vi "Execute Tests.vi"(8 "error in (no error)":errorcluster, 10 "Tests":string[](array[string]), 11 "Execution UI In":refnum<class "Execution UI.lvclass">) -> (0 "error out":errorcluster, 3 "Execution UI Out":refnum<class "Execution UI.lvclass">)   [LabVIEW 2020, in "Execution UI.lvclass"]
uses:
  Execution UI.lvclass
  TypeDefs/Execution State.ctl
  Execution UI.lvclass/Execution UI.ctl
  LUnit Test Suite.lvclass
  C:/git/astemes-lunit/source/Runnable.lvclass
  Framework/Plugin/Plugin.lvclass
  Framework/Test Runner/Test Runner.lvclass
  Result Model by Reference/Result Model by Reference.lvclass
  C:/git/astemes-lunit/source/LUnit Test Suite.lvclass
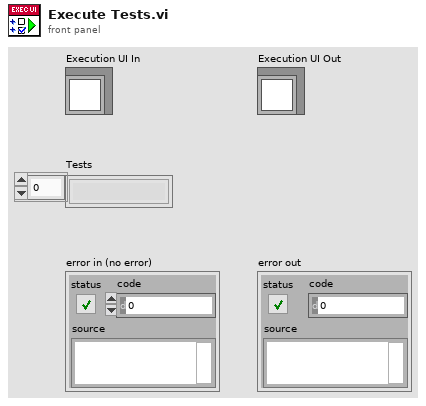
[diagram p1: front panel]
types:
  T1 = typedef "Execution UI.lvclass/Execution State.ctl" = enum16{"Idle", "Running"}
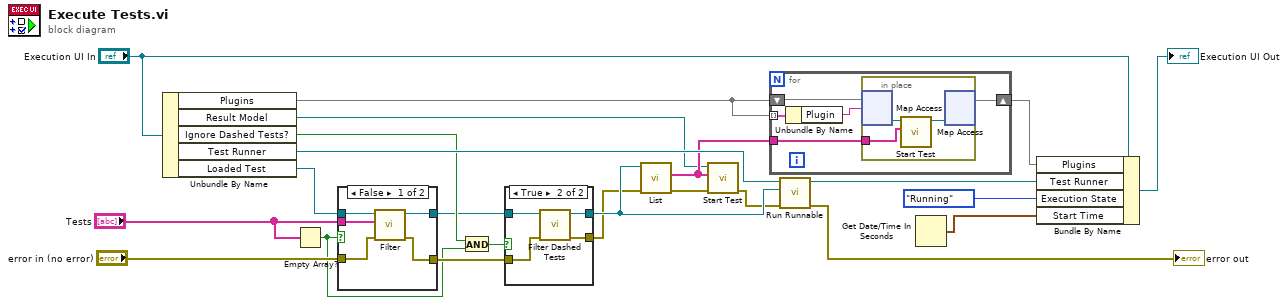
[diagram p0: block diagram]
diagram:
  n1 = Unbundle By Name("Execution UI In") -> ("Plugins"=w7:map{string, refnum<class "Plugin.lvclass">}, "Result Model"=w8:refnum<class "Result Model by Reference.lvclass">, "Ignore Dashed Tests?"=w16:bool, "Test Runner"=w23:refnum<class "Test Runner.lvclass">, "Loaded Test"=w14:refnum<class "LUnit Test Suite.lvclass">)
  n2 = Empty Array?(array="Tests") -> (empty?=w10:bool)
  n3 = case shown="False" w10 {
    tunnel: "error in (no error)" -> [w28 w30]
    tunnel: w14 -> [w27 w29]
    tunnel: [w26 w29] -> w13
    tunnel: "Tests" -> [w25 _]
    tunnel: [w24 w30] -> w11
    frame False {
      n4 = call "Filter.vi"("error in (no error)"=w28, "Selected Runnables"=w25, "LUnit Test Suite In"=w27) -> ("error out"=w24:errorcluster, "LUnit Test Suite Out"=w26:refnum<class "LUnit Test Suite.lvclass">)  [unwired: 7 in]
    }
    frame True {
    }
  }
  n5 = And(x=w16, y=w10) -> (x .and. y?=w15:bool)
  n6 = case shown="True" w15 {
    tunnel: w11 -> [w31 w33]
    tunnel: [w31 w34] -> w5
    tunnel: w13 -> [w32 w35]
    tunnel: [w32 w36] -> w17
    frame False {
    }
    frame True {
      n7 = call "Filter Dashed Tests.vi"("error in (no error)"=w33, "Test Suite"=w35) -> ("error out"=w34:errorcluster, "Filtered Test Suite"=w36:refnum<class "LUnit Test Suite.lvclass">)  [unwired: 8 in]
    }
  }
  n8 = call "List.vi"("error in (no error)"=w5, "LUnit Test Suite In"=w17) -> ("error out"=w20:errorcluster, "List of Runnables"=w19:string[])  [unwired: 8 in]
  n9 = call "Start Test.vi"("error in (no error)"=w20, "Tests"=w19, "Result Model In"=w8) -> ("error out"=w4:errorcluster)  [unwired: 8 in]
  n10 = for {
    tunnel: w19 -> [w38]
    shift-right: [w37] -> w6
    shift-left: w7 -> [w41]
    tunnel: w7 -> [w40] mode=indexing
    n11 = Unbundle By Name(w40) -> ("Plugin"=w39:string)
    n12 = in-place {
      in-place-border: w38 -> [w43]
      n13 = in-place-map #1(w41, w39) -> (w44:refnum<class "Plugin.lvclass">)  [unwired: 1 in, 1 out]
      n14 = call-dynamic "Start Test.vi"("Tests"=w43, "Plugin in"=w44) -> ("Plugin out"=w42:refnum<class "Plugin.lvclass">)  [unwired: 8 in, 1 out]
      n15 = in-place-map #1(w42) -> (w37:map{string, refnum<class "Plugin.lvclass">})  [unwired: 1 in, 2 out]
    }
  }
  n16 = call-dynamic "Run Runnable.vi"("error in (no error)"=w4, "Runnable"=w17, "Test Runner In"=w23) -> ("error out"=→"error out":errorcluster, "Test Runner Out"=w22:refnum<class "Test Runner.lvclass">)  [unwired: 7 in]
  n17 = Get Date/Time In Seconds() -> (seconds since 1Jan1904=w1:timestamp)
  n18 = Bundle By Name(cluster="Execution UI In", "Plugins"=w6, "Test Runner"=w22, "Execution State"=Execution_State."Running", "Start Time"=w1) -> (→"Execution UI Out":refnum<class "Execution UI.lvclass">)
